vi "centroid calcluation.vi"(7 "threshold fraction":sgl, 8 "error in (no error)":errorcluster, 9 "Range":cluster{"Lower value":sgl, "Upper value":sgl}, 10 "Use threshold fraction":bool, 11 "Refnum in":T1) -> (0 "error out":errorcluster, 2 "Numeric":u32, 3 "Centroid":cluster{"X Centroid":sgl, "Y Centroid":sgl})   [LabVIEW 2020]
uses:
  <vilib>/vision/NI_Vision_Development_Module.lvlib
  <vilib>/vision/Image Controls.llb/IMAQ Image.ctl
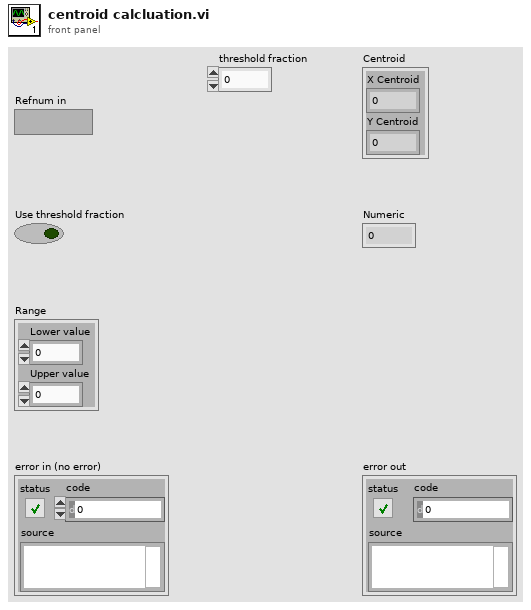
[diagram p1: front panel]
types:
  T1 = typedef "IMAQ Image.ctl" = refnum<image>
  T2 = cluster{"histogram":u32[], "Minimal Value":sgl, "Maximal Value":sgl, "Starting Value":sgl, "Interval Width":sgl, "Mean Value":sgl, "Standard  Variation":sgl, "Area (pixels)":i32}
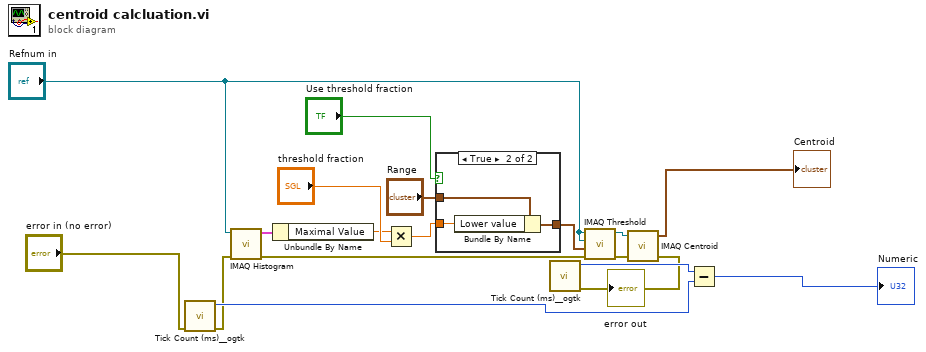
[diagram p0: block diagram]
diagram:
  n1 = call <userlib>:"Tick Count (ms)__ogtk.vi"("error in (no error)"="error in (no error)") -> ("error out"=w14:errorcluster, "millisecond timer value"=w18:u32)  [unwired: 9 in]
  n2 = call "IMAQ Histogram"("error in (no error)"=w14, "Image"="Refnum in") -> ("error out"=w8:errorcluster, "Histogram Report"=w4:T2)  [unwired: 8 in]
  n3 = Unbundle By Name(w4) -> ("Maximal Value"=w6:sgl)
  n4 = Multiply(x=w6, y="threshold fraction") -> (x*y=w12:sgl)
  n5 = case shown="True" "Use threshold fraction" {
    tunnel: [w20 w22] -> w11
    tunnel: "Range" -> [w20 w23]
    tunnel: w12 -> [_ w21]
    frame False {
    }
    frame True {
      n6 = Bundle By Name(cluster=w23, "Lower value"=w21) -> (w22:cluster{"Lower value":sgl, "Upper value":sgl})
    }
  }
  n7 = call "IMAQ Threshold"("error in (no error)"=w8, "Range"=w11, "Image Dst"="Refnum in", "Image Src"="Refnum in") -> ("error out"=w2:errorcluster, "Image Dst Out"=w3:T1)  [unwired: 6 in]
  n8 = call "IMAQ Centroid"("error in (no error)"=w2, "Image"=w3) -> ("error out"=w15:errorcluster, "Centroid"=→"Centroid":cluster{"X Centroid":sgl, "Y Centroid":sgl})  [unwired: 2 in]
  n9 = call <userlib>:"Tick Count (ms)__ogtk.vi"("error in (no error)"=w15) -> ("error out"=→"error out":errorcluster, "millisecond timer value"=w17:u32)  [unwired: 9 in]
  n10 = Subtract(x=w17, y=w18) -> (x-y=→"Numeric":u32)
